vi "temp create RCVR files.vi"(10 "Base File Path":path, 11 "Location":string="RCVR 1" caption="Name of RCVR") -> (1 "error out":errorcluster, 2 "refnum out":refnum<file>, 3 "Name of file out":string)   [LabVIEW 2012]
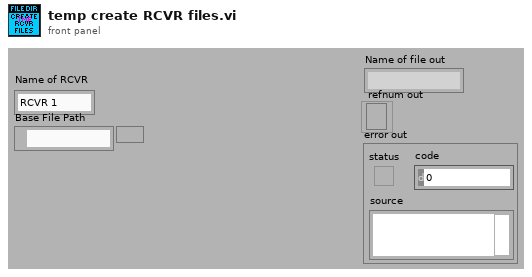
[diagram p1: front panel]
types:
  T1 = enum16{"open", "replace", "create", "open or create", "replace or create", "replace or create with confirmation"}
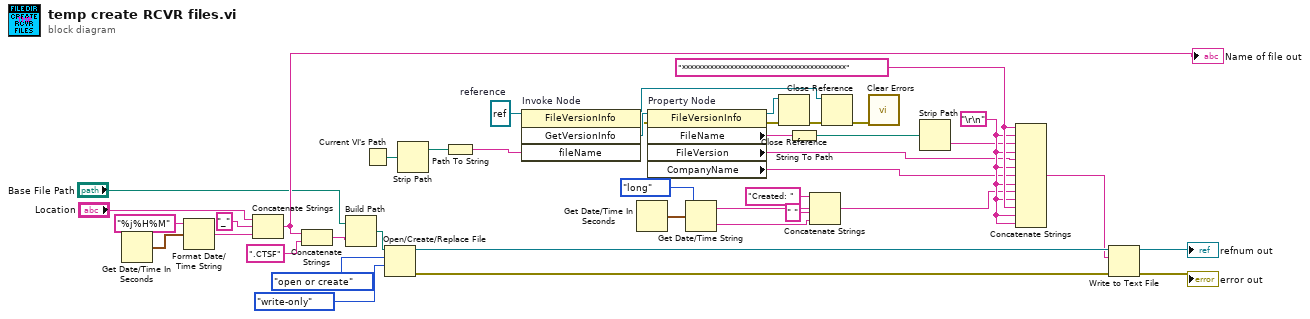
[diagram p0: block diagram]
diagram:
  w1 = refnum<k24> refnum  # reference
  w27 = "\r\n"
  w28 = "*****************************************" ("string")
  n1 = Get Date/Time In Seconds() -> (seconds since 1Jan1904=w2:timestamp)
  n2 = Format Date/Time String(time format string (%c)="%j%H%M", seconds (now)=w2) -> (date/time string=w34:string)  [unwired: 1 in]
  n3 = Concatenate Strings("Location", "_" ("string"), w34) -> (w42:string)
  "Name of file out" <- w42
  n4 = Concatenate Strings(w42, ".CTSF" ("string")) -> (w31:string)
  n5 = Build Path(base path="Base File Path", name or relative path=w31) -> (appended path=w36:path)
  n6 = Current VI's Path() -> (path=w17:path)
  n7 = Open/Create/Replace File(file path (use dialog)=w36, operation (0:open)=T1."open or create", access (0:read/write)=enum16{"read/write", "read-only", "write-only"}."write-only") -> (refnum out=w30:refnum<file>, error out=w29:errorcluster)  [unwired: 3 in, 1 out]
  n8 = Strip Path(path=w17) -> (stripped path=w16:path)  [unwired: 1 out]
  n9 = Path To String(path=w16) -> (string=w15:string)
  n10 = invoke on="Invoke Node" class="FileVersionInfo" method="GetVersionInfo"(reference=w1, "fileName"=w15) -> (reference out=w9:refnum<k24>, error out=w13:errorcluster, "GetVersionInfo"=w14:refnum<k24>)  [unwired: 2 in, 1 out]
  n11 = Get Date/Time In Seconds() -> (seconds since 1Jan1904=w20:timestamp)
  n12 = property on="Property Node" class="FileVersionInfo"(reference=w14, error in=w13) -> (reference out=w12:refnum<k24>, error out=w11:errorcluster, "FileName"=w6:string, "FileVersion"=w8:string, "CompanyName"=w7:string)
  n13 = Get Date/Time String(date format (0)=enum16{"short", "long", "abbreviated"}."long", seconds (now)=w20) -> (date string=w23:string, time string=w25:string)  [unwired: 1 in]
  n14 = Close Reference(reference=w12, error in (no error)=w11) -> (error out=w10:errorcluster)
  n15 = String To Path(string=w6) -> (path=w5:path)
  n16 = Concatenate Strings("Created: " ("string"), w23, " " ("string"), w25) -> (w26:string)
  n17 = Close Reference(reference=w9, error in (no error)=w10) -> (error out=w18:errorcluster)
  n18 = call <vilib>:"Clear Errors.vi"("error in (no error)"=w18) -> ()  [unwired: 6 in, 1 out]
  n19 = Strip Path(path=w5) -> (name=w4:string)  [unwired: 1 out]
  n20 = Concatenate Strings(w28, w27, w4, w27, w8, w27, w7, w27, w26, w27, w28, w27, w27) -> (w19:string)
  n21 = Write to Text File(file (use dialog)=w30, text=w19, error in=w29) -> (refnum out=→"refnum out":refnum<file>, error out=→"error out":errorcluster)  [unwired: 1 in, 1 out]
